vi "Inject Attribute List.vi"(6 "Attributes Ref":refnum<data-value>, 8 "error in (no error)":errorcluster, 11 "Stop Bug Remover in":refnum<class "Stop Tire Shine Foam.lvclass">) -> (0 "error out":errorcluster, 3 "Stop Bug Remover out":refnum<class "Stop Tire Shine Foam.lvclass">)   [LabVIEW 2019, in "Stop Tire Shine Foam.lvclass"]
uses:
  <vilib>/gpm_packages/@cs/Car-wash/Source/Process Steps/Stop Tire Shine Foam/Stop Tire Shine Foam.lvclass
  <vilib>/gpm_packages/@cs/lookup-table/Source/LookupTable/LookupTable.lvclass
  <vilib>/gpm_packages/@cs/lookup-table/Source/LookupTable/LookupTable.lvclass/LookupTable.ctl
  <vilib>/gpm_packages/@cs/Car-wash/Source/Process Steps/Stop Tire Shine Foam/Stop Tire Shine Foam.lvclass/Stop Tire Shine Foam.ctl
  29fbb1c8-51b9-41f4-9131-374242a790d5.vi
  <vilib>/gpm_packages/@cs/lookup-table/Source/LookupTable/Read Table Reference.vi
  29fbb1c8-51b9-41f4-9131-374242a790d5.vi/9a41755b-4497-47d5-9d6c-bec36d2adcc2.vi
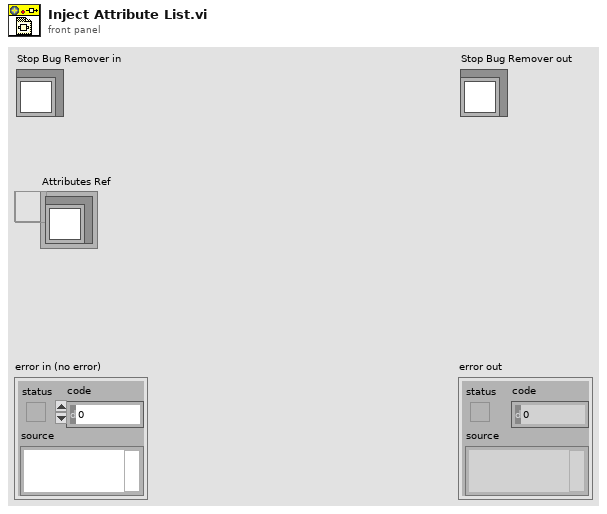
[diagram p1: front panel]
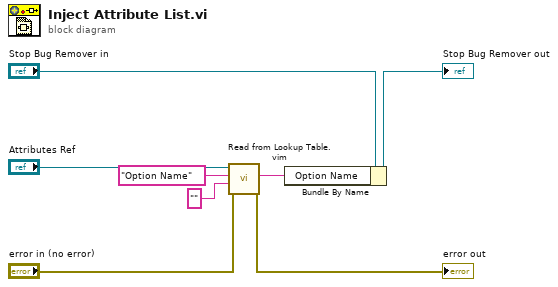
[diagram p0: block diagram]
diagram:
  n1 = call "Read from Lookup Table.vim"("error in (no error)"="error in (no error)", "Type"="", "Item Name"="Option Name", "LookupTable Reference"="Attributes Ref") -> ("error out"=→"error out":errorcluster, "Value"=w6:string)  [unwired: 4 in, 2 out]
  n2 = Bundle By Name(cluster="Stop Bug Remover in", "Option Name"=w6) -> (→"Stop Bug Remover out":refnum<class "Stop Tire Shine Foam.lvclass">)
